vi "Image Pixel Adjustment - SubVI.vi"(8 "error in":errorcluster, 9 "Set to Maximum":bool, 10 "Set to 512 x 300":bool, 11 "Set to AOI":bool) -> (0 "Pixels Out":i32[](array[numeric]), 1 "Error Out (no error)":errorcluster)   [LabVIEW 2014]
uses:
  Glimpse-master/Microscope plugins/ixon1024/HAL camera parameters important.ctt
  Glimpse-master/Microscope plugins/ixon1024/ixon readout settings.ctl
  Glimpse-master/Microscope plugins/ixon1024/andor acquisition mode.ctl
  Initilize Globals.vi
panel:
  in  "Camera Parameters (important)":T1={"Exposure Time (sec)"=0.1, "EM CCD Gain"=230, "Readout Settings"={"Acquisition Mode"=enum."Single Scan", "Pixel Rate"=enum."EM CCD 1 Mhz 16 bits", "High Capacity?"=FALSE, "V Shift Speed (us/row)"=enum."3.3  (not reccommended)", "V Shift Amplitude"=enum."+1", "Preamp Gain"=enum."2.4", "Trigger Mode"=0}, "Image Size"={"H Bin"=1, "V Bin"=1, "Left"=1, "Top"=1, "Right"=512, "Bottom"=512}, "Shutter"=0} {"Shutter" items=["Auto", "Stay Open", "Always Closed"]; "Readout Settings"."Trigger Mode" items=["Internal", "External"]; "EM CCD Gain" scale=1.0..300.0; "Exposure Time (sec)" scale=0.001..10.0 scale format="%#_1g"}
  # "Camera: Andor iXon"
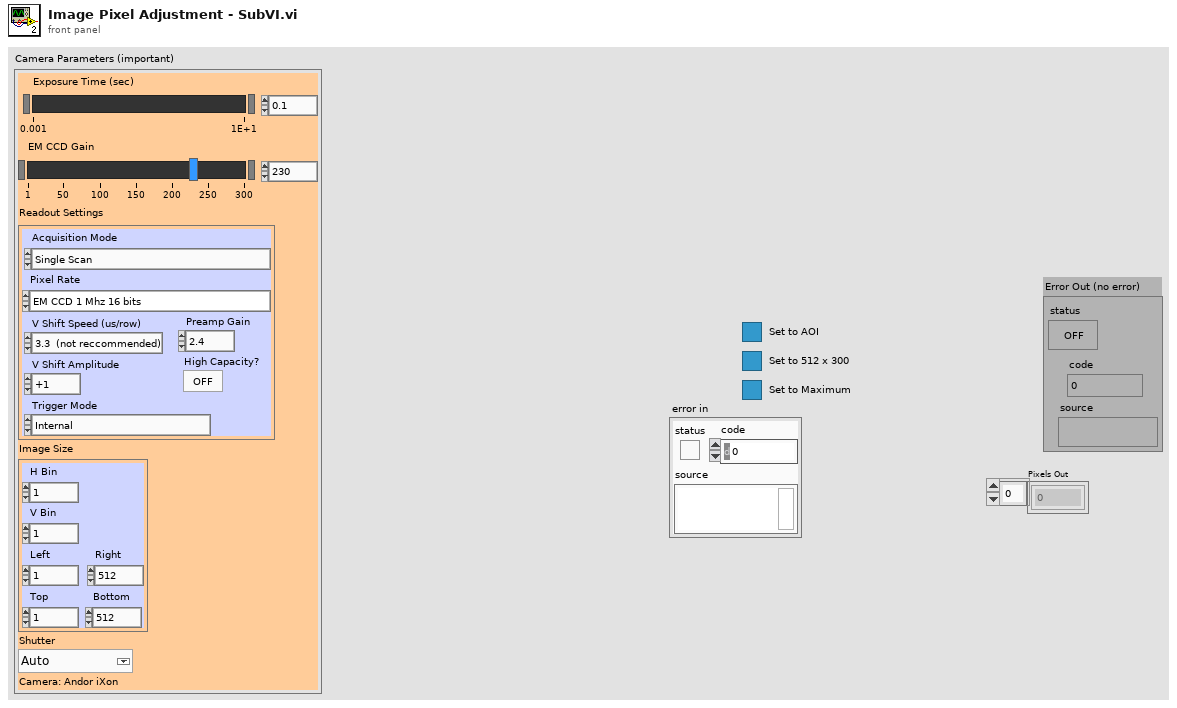
[diagram p1: front panel]
types:
  T1 = typedef "HAL camera parameters important.ctt" = cluster{"Exposure Time (sec)":sgl, "EM CCD Gain":u16, "Readout Settings":T2, "Image Size":cluster{"H Bin":i32, "V Bin":i32, "Left":i32, "Top":i32, "Right":i32, "Bottom":i32}, "Shutter":i32}
  T2 = typedef "ixon readout settings.ctl" = cluster{"Acquisition Mode":T3, "Pixel Rate":enum16{"EM CCD 10 Mhz 14 bits", "EM CCD 5 Mhz 14 bits", "EM CCD 3 Mhz 14 bits", "EM CCD 1 Mhz 16 bits", "Standard CCD 3 Mhz 14 bits", "Standard CCD 1 Mhz 16 bits"}, "High Capacity?":bool, "V Shift Speed (us/row)":enum16{"0.9 (not reccommended)", "1.7  (not reccommended)", "3.3  (not reccommended)", "6.5", "12.9"}, "V Shift Amplitude":enum16{"normal", "+1", "+2", "+3", "+4"}, "Preamp Gain":enum16{"1.0", "2.4", "5.0"}, "Trigger Mode":u32}
  T3 = typedef "andor acquisition mode.ctl" = enum16{"(do not use)", "Single Scan", "Accumulate", "Kinetics", "Fast Kinetics", "Kinetics Run till Abort", "Frame Transfer", "Frame Transfer Run till Abort", "(do not use) ", "Time Delayed Integration"}
  T4 = cluster{"H Bin":dbl, "V Bin":dbl, "Left":dbl, "Right":dbl, "Top":dbl, "Bottom":dbl}
  T5 = typedef "ROI Descriptor" = cluster{"Global Rectangle":i32[], "Contours":cluster{"ID":enum32{"External", "Internal"}, "Type":u32, "Coordinates":i32[]}[]}
  T6 = cluster{"H Pixels":dbl, "V Pixels":dbl, "Minimum Temperature":dbl, "Maximum Temperature":dbl}
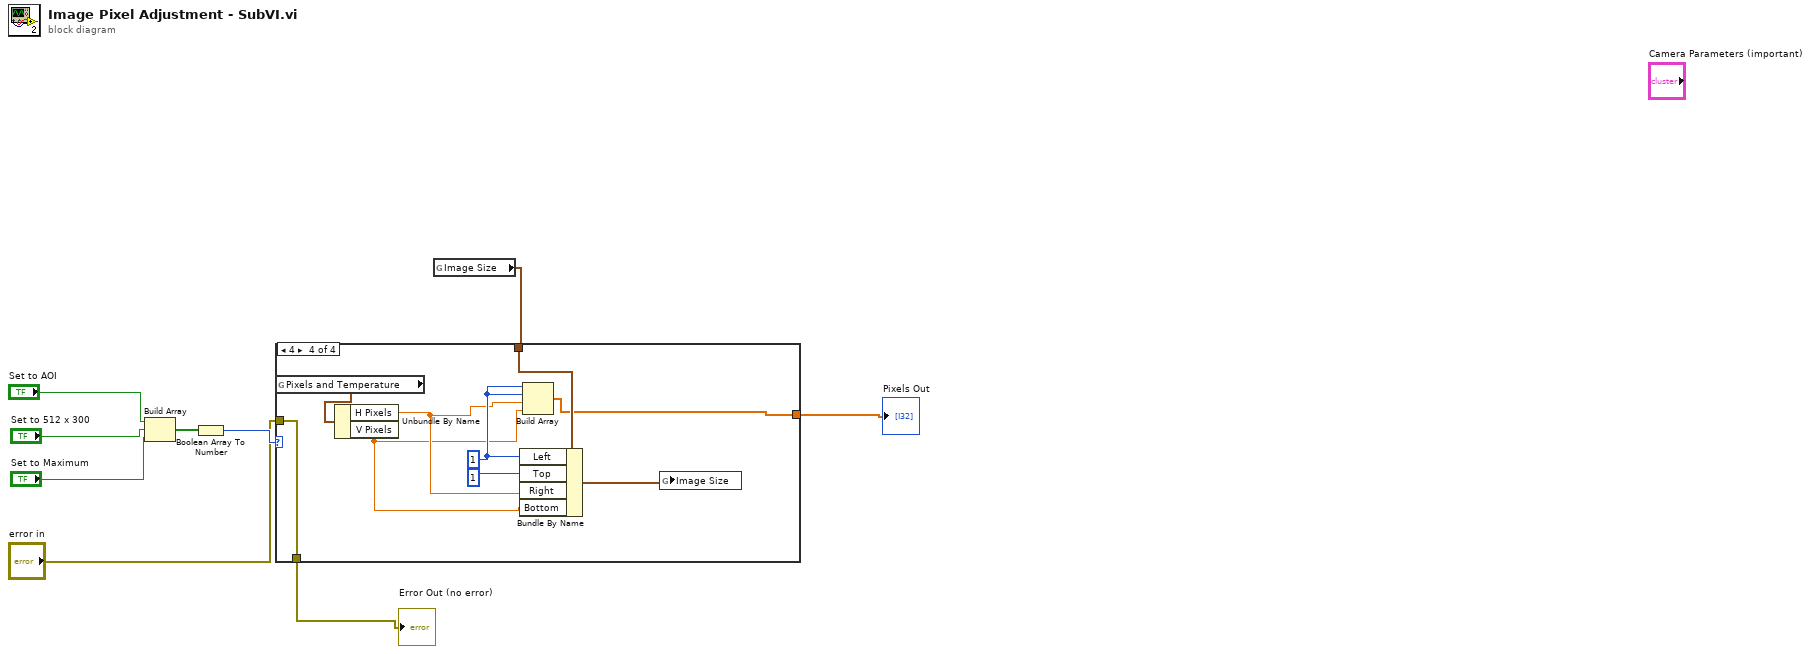
[diagram p0: block diagram]
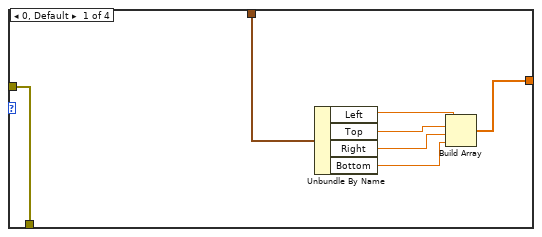
[diagram p2: hidden frame]
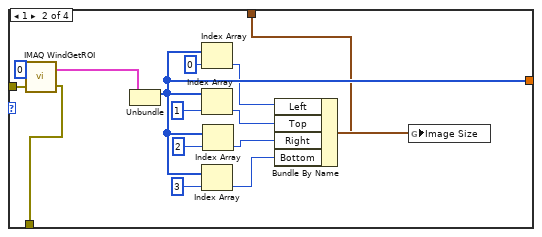
[diagram p3: hidden frame]
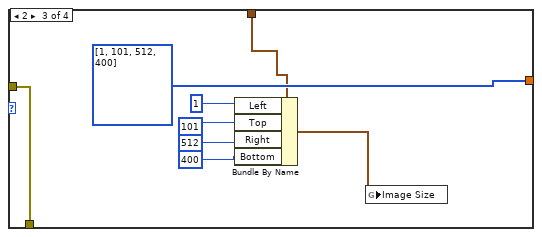
[diagram p4: hidden frame]
diagram:
  n1 = Build Array("Set to AOI", "Set to 512 x 300", "Set to Maximum") -> (w6:bool[])
  n2 = Boolean Array To Number(Boolean array=w6) -> (number=w5:u32)
  n3 = global read "Initilize Globals.vi" "Image Size"() -> (w2:T4)
  n4 = case shown="4" w5 {
    tunnel: "error in" -> [w16 w31 w39 w48]
    tunnel: [w10 w24 i32[] [1, 101, 512, 400] ("Global Rectangle") w40] -> w1
    tunnel: [w16 w29 w39 w48] -> w3
    tunnel: w2 -> [w11 w17 w32 w45]
    frame 0, Default {
      n5 = Unbundle By Name(w11) -> ("Left"=w12:dbl, "Top"=w13:dbl, "Right"=w14:dbl, "Bottom"=w15:dbl)
      n6 = Build Array(w12, w13, w14, w15) -> (w10:dbl[])
    }
    frame 1 {
      n7 = call "IMAQ WindGetROI"("Window Number (0...15)"=0, "error in (no error)"=w31) -> ("ROI Descriptor"=w30:T5, "error out"=w29:errorcluster)  [unwired: 3 out]
      n8 = Unbundle(w30) -> ("Global Rectangle"=w24:i32[])  [unwired: 1 out]
      n9 = Index Array(array=w24, index=0) -> (element=w22:i32)
      n10 = Index Array(array=w24, index=1) -> (element=w21:i32)
      n11 = Index Array(array=w24, index=3) -> (element=w19:i32)
      n12 = Index Array(array=w24, index=2) -> (element=w20:i32)
      n13 = Bundle By Name(cluster=w17, "Left"=w22, "Top"=w21, "Right"=w20, "Bottom"=w19) -> (w23:T4)
      n14 = global write "Initilize Globals.vi" "Image Size"(w23) -> ()
    }
    frame 2 {
      n15 = Bundle By Name(cluster=w32, "Left"=1, "Top"=101, "Right"=512, "Bottom"=400) -> (w36:T4)
      n16 = global write "Initilize Globals.vi" "Image Size"(w36) -> ()
    }
    frame 4 {
      w43 = 1 ("Left")
      n17 = global read "Initilize Globals.vi" "Pixels and Temperature"() -> (w44:T6)
      n18 = Unbundle By Name(w44) -> ("H Pixels"=w42:dbl, "V Pixels"=w41:dbl)
      n19 = Bundle By Name(cluster=w45, "Left"=w43, "Top"=1, "Right"=w42, "Bottom"=w41) -> (w47:T4)
      n20 = Build Array(w43, w43, w42, w41) -> (w40:dbl[])
      n21 = global write "Initilize Globals.vi" "Image Size"(w47) -> ()
    }
  }
  "Error Out (no error)" <- w3
  "Pixels Out" <- w1
